vi "CodigoLabView 2.vi"() -> ()   [LabVIEW 2025]
uses:
  <vilib>/Instr/_visa.llb/VISA Configure Serial Port (Instr).vi
panel:
  out "Estado 4":string
  out "rele 4":string
  out "Rele 4":bool
  in  "Relé N°4":bool
  out "Estado 3":string
  out "rele 3":string
  out "Rele 3":bool
  in  "Relé N°3":bool
  out "Estado 2":string
  out "rele 2":string
  out "Rele 2":bool
  in  "Relé N°2":bool
  out "Estado 1":string
  out "rele 1":string
  out "Rele 1":bool
  in  "Relé N°1":bool
  out "Serial Settings:Number of Bytes at Serial Port":u32
  out "error out 2":errorcluster
  out "Enviando":string
  out "error out":errorcluster
  in  "VISA resource name":refnum<visa-resource-name>
  in  "stop":bool
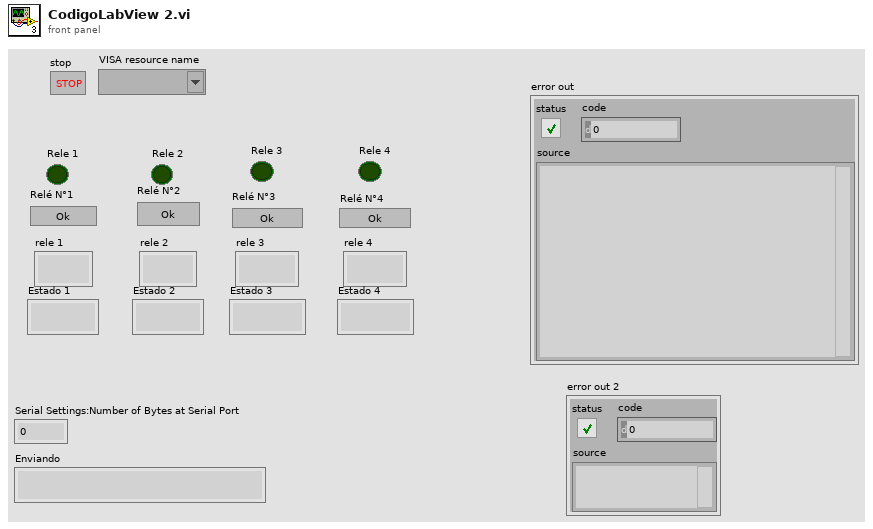
[diagram p1: front panel]
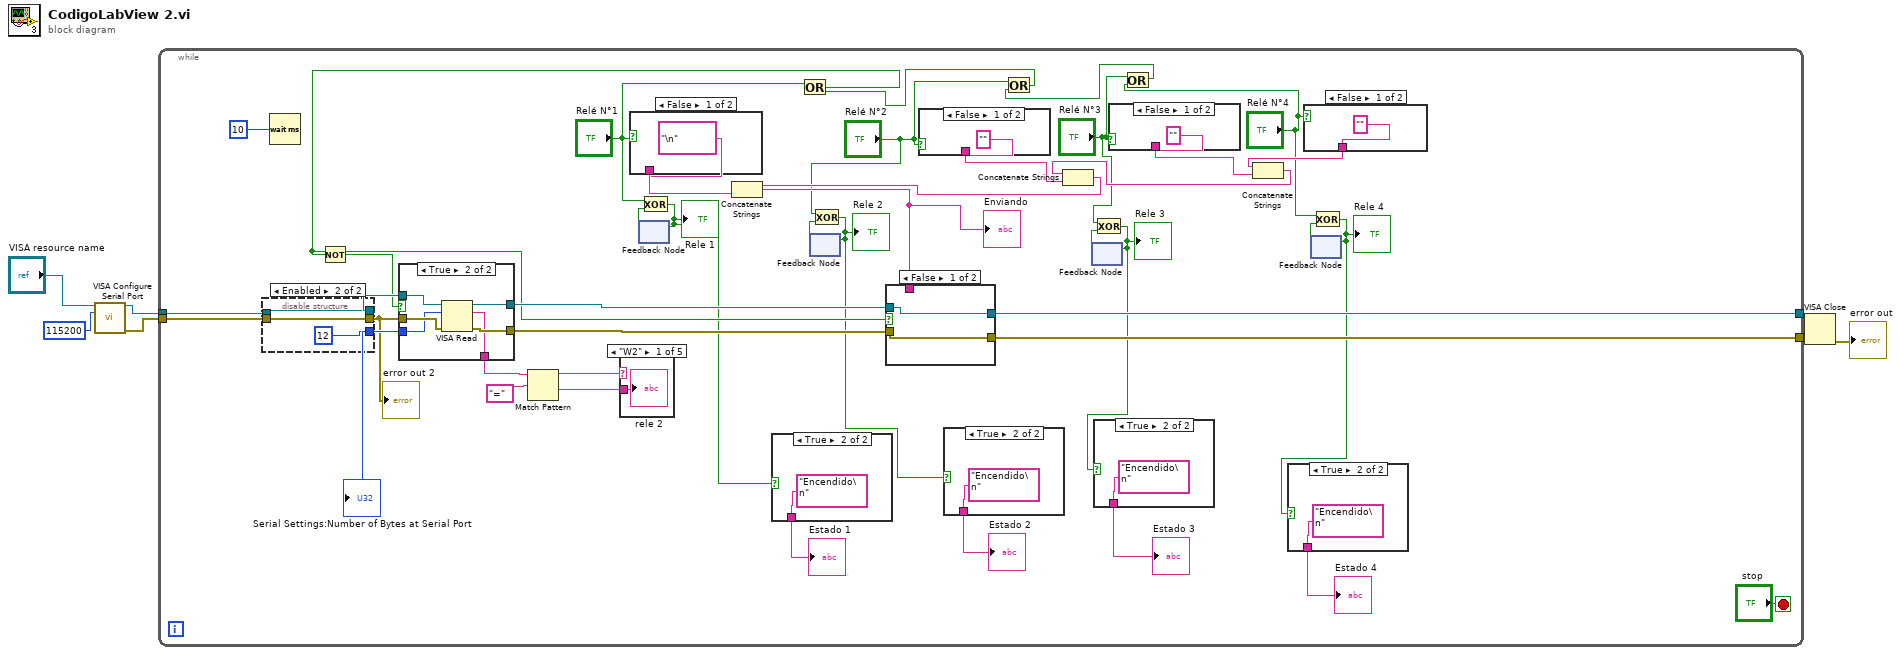
[diagram p0: block diagram]
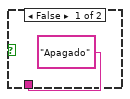
[diagram p2: hidden frame]
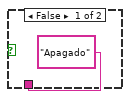
[diagram p3: hidden frame]
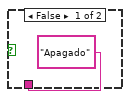
[diagram p4: hidden frame]
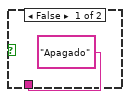
[diagram p5: hidden frame]
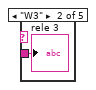
[diagram p6: hidden frame]
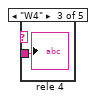
[diagram p7: hidden frame]
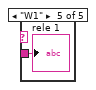
[diagram p9: hidden frame]
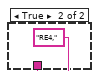
[diagram p10: hidden frame]
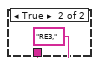
[diagram p11: hidden frame]
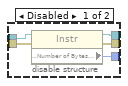
[diagram p12: hidden frame]
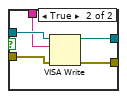
[diagram p14: hidden frame]
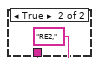
[diagram p15: hidden frame]
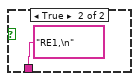
[diagram p16: hidden frame]
diagram:
  n1 = call-poly "VISA Configure Serial Port"("VISA resource name"="VISA resource name", "baud rate (9600)"=u32 115200) -> ("VISA resource name out"=w7:refnum<visa-resource-name>, "error out"=w1:errorcluster)  [unwired: 12 in]
  n2 = while {
    tunnel: w7 -> [w48]
    tunnel: [w45] -> w6
    tunnel: w1 -> [w47]
    tunnel: [w44] -> w5
    stop <- "stop" stop-if-true
    n3 = disable-structure shown="Enabled" {
      disable-tunnel: w48 -> [w70 w73]
      disable-tunnel: w47 -> [w69 w72]
      disable-tunnel: [w68 w73] -> w41
      disable-tunnel: [w67 u32 12 ("Bytes at Port")] -> w40
      disable-tunnel: [w66 w72] -> w39
      frame Disabled {
        n4 = property class="Instr"(reference=w70, error in=w69) -> (reference out=w68:refnum<visa-resource-name>, error out=w66:errorcluster, "Serial Settings:Number of Bytes at Serial Port"=w67:u32)
      }
      frame Enabled {
      }
    }
    "error out 2" <- w39
    "Serial Settings:Number of Bytes at Serial Port" <- w40
    n5 = Wait (ms)(milliseconds to wait=u32 10) -> ()  [unwired: 1 out]
    n6 = case shown="False" "Relé N°1" {
      tunnel: ["\n" "RE1,\n"] -> w46
      frame False {
      }
      frame True {
      }
    }
    n7 = feedback #1() -> (w23:bool)  [unwired: 1 in]
    n8 = Exclusive Or(1:w23, 2:"Relé N°1") -> (0:w8:bool)
    "Rele 1" <- w8
    n9 = feedback-in #1(w8) -> ()
    n10 = case shown="True" w8 {
      tunnel: ["Apagado" "Encendido\n"] -> w12
      frame False {
      }
      frame True {
      }
    }
    "Estado 1" <- w12
    n11 = feedback #2() -> (w22:bool)  [unwired: 1 in]
    n12 = Exclusive Or(1:w22, 2:"Relé N°2") -> (0:w9:bool)
    "Rele 2" <- w9
    n13 = feedback-in #2(w9) -> ()
    n14 = case shown="False" "Relé N°2" {
      tunnel: ["" "RE2,"] -> w30
      frame False {
      }
      frame True {
      }
    }
    n15 = case shown="True" w9 {
      tunnel: ["Apagado" "Encendido\n"] -> w13
      frame False {
      }
      frame True {
      }
    }
    "Estado 2" <- w13
    n16 = feedback #3() -> (w20:bool)  [unwired: 1 in]
    n17 = Exclusive Or(1:w20, 2:"Relé N°3") -> (0:w10:bool)
    "Rele 3" <- w10
    n18 = feedback-in #3(w10) -> ()
    n19 = case shown="True" w10 {
      tunnel: ["Apagado" "Encendido\n"] -> w14
      frame False {
      }
      frame True {
      }
    }
    "Estado 3" <- w14
    n20 = case shown="False" "Relé N°3" {
      tunnel: ["" "RE3,"] -> w32
      frame False {
      }
      frame True {
      }
    }
    n21 = Or(x="Relé N°3", y="Relé N°4") -> (x .or. y?=w35:bool)
    n22 = Or(x="Relé N°2", y=w35) -> (x .or. y?=w34:bool)
    n23 = Or(x="Relé N°1", y=w34) -> (x .or. y?=w37:bool)
    n24 = Not(x=w37) -> (.not. x?=w38:bool)
    n25 = case shown="True" w38 {
      tunnel: [w75 w81] -> w43
      tunnel: [w74 w80] -> w42
      tunnel: w39 -> [w74 w79]
      tunnel: w41 -> [w75 w78]
      tunnel: w40 -> [_ w77]
      tunnel: [_ w76] -> w27
      frame False {
      }
      frame True {
        n26 = VISA Read(VISA resource name=w78, byte count=w77, error in (no error)=w79) -> (VISA resource name out=w81:refnum<visa-resource-name>, read buffer=w76:string, error out=w80:errorcluster)  [unwired: 1 out]
      }
    }
    n27 = Match Pattern(string=w27, regular expression="=") -> (before substring=w25:string, after substring=w16:string)  [unwired: 1 in, 2 out]
    n28 = case shown="\"W2\"" w25 {
      tunnel: w16 -> [w58 w59 w60 _ w61]
      frame "W2" {
        "rele 2" <- w58
      }
      frame "W3" {
        "rele 3" <- w59
      }
      frame "W4" {
        "rele 4" <- w60
      }
      frame "False", Default {
      }
      frame "W1" {
        "rele 1" <- w61
      }
    }
    n29 = case shown="False" "Relé N°4" {
      tunnel: ["" "RE4,"] -> w33
      frame False {
      }
      frame True {
      }
    }
    n30 = Concatenate Strings(w33, w32) -> (w31:string)
    n31 = Concatenate Strings(w31, w30) -> (w29:string)
    n32 = Concatenate Strings(w29, w46) -> (w28:string)
    "Enviando" <- w28
    n33 = case shown="False" w37 {
      tunnel: [w83 w88] -> w45
      tunnel: [w82 w87] -> w44
      tunnel: w43 -> [w83 w86]
      tunnel: w42 -> [w82 w85]
      tunnel: w28 -> [_ w84]
      frame False {
      }
      frame True {
        n34 = VISA Write(VISA resource name=w86, write buffer=w84, error in (no error)=w85) -> (VISA resource name out=w88:refnum<visa-resource-name>, error out=w87:errorcluster)  [unwired: 1 out]
      }
    }
    n35 = feedback #4() -> (w19:bool)  [unwired: 1 in]
    n36 = Exclusive Or(1:w19, 2:"Relé N°4") -> (0:w11:bool)
    "Rele 4" <- w11
    n37 = case shown="True" w11 {
      tunnel: ["Apagado" "Encendido\n"] -> w15
      frame False {
      }
      frame True {
      }
    }
    "Estado 4" <- w15
    n38 = feedback-in #4(w11) -> ()
  }
  n39 = VISA Close(VISA resource name=w6, error in (no error)=w5) -> (error out=→"error out":errorcluster)
